vi "HardwareQueueCreate.vi"(2 "error in (no error)":errorcluster) -> (0 "HardwareError":errorcluster, 1 "HardwareQueue":refnum<queue>)   [LabVIEW 2017]
uses:
  HardwareQueueCluster.ctl
  hardwareMessage.ctl
panel:
  in  "QueueName":string
  in  "HardwareQueueCluster":T1
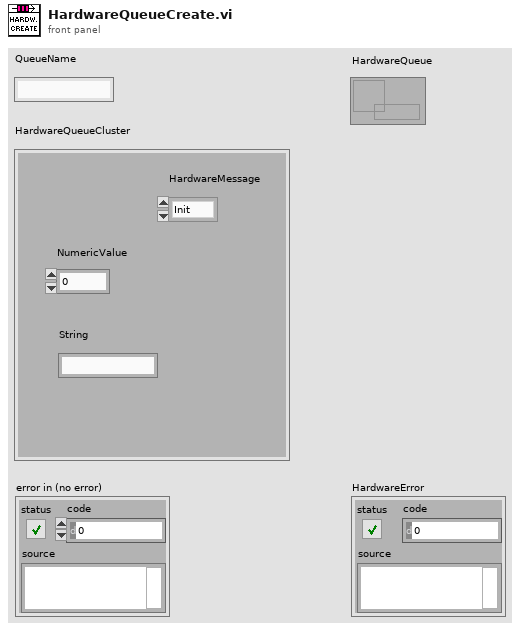
[diagram p1: front panel]
types:
  T1 = typedef "HardwareQueueCluster.ctl" = cluster{"HardwareMessage":T2, "NumericValue":dbl, "String":string}
  T2 = typedef "hardwareMessage.ctl" = enum16{"Init", "MeasureChannel", "CloseDevice", "Error", "Halt", "SetPhysChannel1", "SetPhysChannel2", "SetPhysChannel3"}
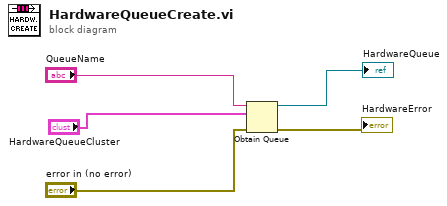
[diagram p0: block diagram]
diagram:
  n1 = Obtain Queue(name (unnamed)="QueueName", element data type="HardwareQueueCluster", error in (no error)="error in (no error)") -> (queue out=→"HardwareQueue":refnum<queue>, error out=→"HardwareError":errorcluster)  [unwired: 2 in, 1 out]
